vi "LVClasse_SurfaceFloatWithPupil Write SurfaceFloatWithPupil.vi"(8 "error in (no error)":errorcluster, 10 "SurfaceFloatWithPupil":i32, 11 "SurfaceFloatWithPupil in":refnum<class "SurfaceFloatWithPupil.lvclass">) -> (0 "error out":errorcluster, 3 "SurfaceFloatWithPupil out":refnum<class "SurfaceFloatWithPupil.lvclass">)   [LabVIEW 2020, in "SurfaceFloatWithPupil.lvclass"]
uses:
  SurfaceFloatWithPupil.lvclass
  SurfaceFloatWithPupil.lvclass/SurfaceFloatWithPupil.ctl
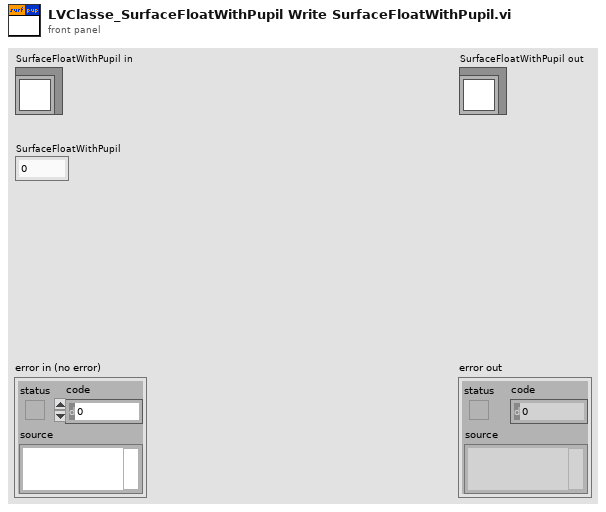
[diagram p1: front panel]
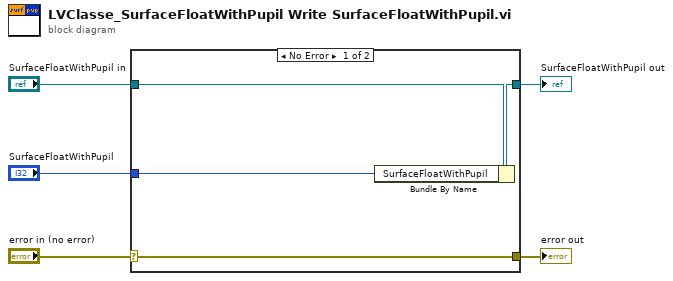
[diagram p0: block diagram]
diagram:
  n1 = case shown="No Error" "error in (no error)" {
    selector: "error in (no error)" -> [w9 w10]
    tunnel: [w9 w10] -> w4
    tunnel: [w7 w11] -> w2
    tunnel: "SurfaceFloatWithPupil in" -> [w8 w11]
    tunnel: "SurfaceFloatWithPupil" -> [w6 _]
    frame No Error {
      n2 = Bundle By Name(cluster=w8, "SurfaceFloatWithPupil"=w6) -> (w7:refnum<class "SurfaceFloatWithPupil.lvclass">)
    }
    frame Error {
    }
  }
  "error out" <- w4
  "SurfaceFloatWithPupil out" <- w2
